vi "file2numden.vi"(11 "File Path":path) -> (0 "Denominator":dbl[](array[numeric]), 1 "Numerator":dbl[](array[numeric]), 3 "FilterLength":i32)   [LabVIEW 2010, in "KevLib01.lvlib"]
uses:
  KevLib01.lvlib
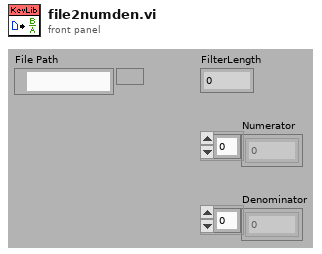
[diagram p1: front panel]
types:
  T1 = enum16{"open", "replace", "create", "open or create", "replace or create", "replace or create with confirmation"}
  T2 = enum16{"deny read/write", "deny write-only", "deny none"}
  T3 = enum16{"big-endian, network order", "native, host order", "little-endian"}
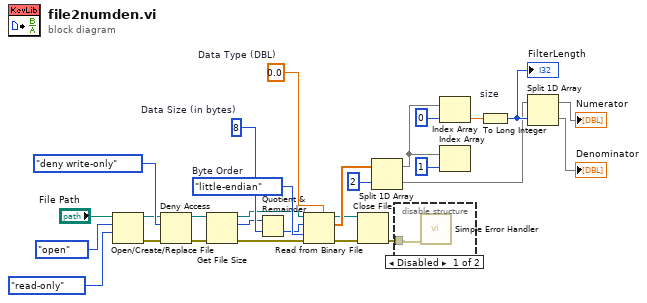
[diagram p0: block diagram]
diagram:
  w13 = T3."little-endian"  # Byte Order
  w11 = i64 8  # Data Size (in bytes)
  w10 = 0.0  # Data Type (DBL)
  n1 = Open/Create/Replace File(file path (use dialog)="File Path", operation (0:open)=T1."open", access (0:read/write)=enum16{"read/write", "read-only", "write-only"}."read-only") -> (refnum out=w15:refnum<file>, error out=w14:errorcluster)  [unwired: 1 in, 3 out]
  n2 = Deny Access(4:w14, 6:T2."deny write-only" ("deny mode (0:deny read/write)"), 7:w15) -> (0:w16:errorcluster, 3:w17:refnum<file>)
  n3 = Get File Size(file=w17, error in=w16) -> (refnum out=w4:refnum<file>, size (in bytes)=w7:i64, 0:w8:errorcluster)
  n4 = Quotient & Remainder(x=w7, y=w11) -> (floor(x/y)=w12:i64)  [unwired: 1 out]
  n5 = Read from Binary File(5:w10, 8:w8, 9:w13, 10:w12, 11:w4) -> (0:w6:errorcluster, 2:w20:dbl[], 3:w5:refnum<file>)  [unwired: 2 out]
  n6 = Close File(refnum=w5, error in=w6) -> (error out=w1:errorcluster)  [unwired: 1 out]
  n7 = Split 1D Array(array=w20, index=2) -> (first subarray=w22:dbl[], second subarray=w24:dbl[])
  n8 = disable-structure shown="Disabled" {
    disable-tunnel: w1 -> [w29 _]
    frame Disabled {
      n9 = call <vilib>:"Simple Error Handler.vi"("error in (no error)"=w29) -> ()  [unwired: 4 in, 5 out]
    }
    frame Enabled {
    }
  }
  n10 = Index Array(array=w22, index=0) -> (element=w23:dbl)
  n11 = Index Array(array=w22, index=1) -> ()  [unwired: 1 out]
  n12 = To Long Integer "size"(number=w23) -> (32bit integer=w26:i32)
  "FilterLength" <- w26
  n13 = Split 1D Array(array=w24, index=w26) -> (first subarray=→"Numerator":dbl[], second subarray=→"Denominator":dbl[])
